vi "Compression Logic.vi"(0 "Tick #":dbl=373.0) -> (7 "Pivot Setpoint":dbl=12.0)   [LabVIEW 2025]
uses:
  <vilib>/Rock Robotics/WPI/DriverStation/WPI_DriverStationRobotMode2.ctl
panel:
  in  "Min Shot":dbl=12.0
  in  "Tick/step # Auto":dbl=7.0
  in  "Tick/step Teleop":dbl=7.0
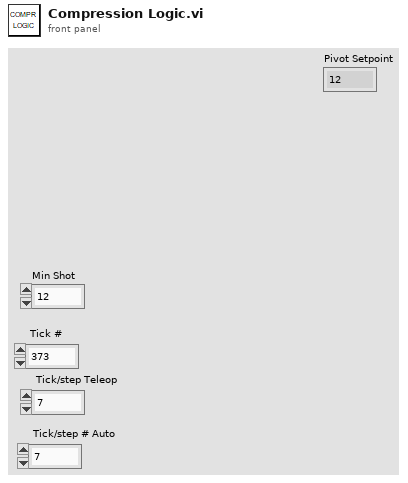
[diagram p1: front panel]
types:
  T1 = typedef "WPI_DriverStationRobotMode2.ctl" = enum16{"Autonomous Disabled", "Autonomous Enabled", "Teleop Disabled", "Teleop Enabled", "Disconnected", "Finish", "Test Disabled", "Test Enabled", "Emergency Stopped"}
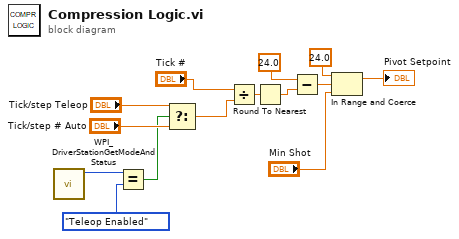
[diagram p0: block diagram]
diagram:
  n1 = call <vilib>:"WPI_DriverStationGetModeAndStatus.vi"() -> ("Robot Mode"=w12:T1)  [unwired: 10 in, 1 out]
  n2 = Equal?(x=w12, y=WPI_DriverStationRobotMode2."Teleop Enabled") -> (x = y?=w10:bool)
  n3 = Select(t="Tick/step Teleop", s=w10, f="Tick/step # Auto") -> (s? t:f=w8:dbl)
  n4 = Divide(x="Tick #", y=w8) -> (x/y=w7:dbl)
  n5 = Round To Nearest(number=w7) -> (nearest integer value=w6:dbl)
  n6 = Subtract(x=24.0, y=w6) -> (x-y=w4:dbl)
  n7 = In Range and Coerce(upper limit=24.0, x=w4, lower limit="Min Shot") -> (coerced(x)=→"Pivot Setpoint":dbl)  [unwired: 1 out]
